vi "MapPositionSend.vi"(8 "error in (no error)":errorcluster caption="错误输入（无错误）", 10 "MapPosition":T1, 11 "CoordinatorState输入":refnum<class "CoordinatorState.lvclass">) -> (0 "error out":errorcluster caption="错误输出", 3 "Process State out":refnum<class "State Actor.lvclass">)   [LabVIEW 2014, in "States.lvlib" / "CoordinatorState.lvclass"]
uses:
  CoordinatorState.lvclass
  <vilib>/NI/Actors/State Actor/State Actor/State Actor.lvclass
  CoordinatorState.lvclass/CoordinatorState.ctl
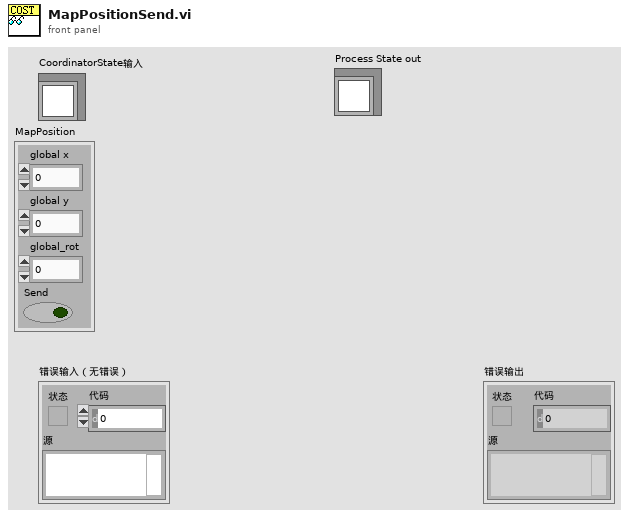
[diagram p1: front panel]
types:
  T1 = cluster{"global x":dbl, "global y":dbl, "global_rot":dbl, "Send":bool}
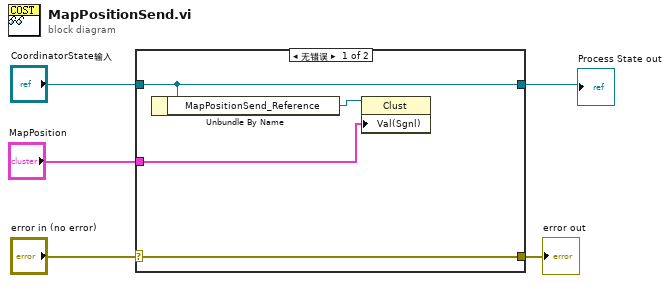
[diagram p0: block diagram]
diagram:
  n1 = case shown="无错误" "error in (no error)" {
    selector: "error in (no error)" -> [w9 w10]
    tunnel: [w9 w10] -> w4
    tunnel: [w8 w11] -> w1
    tunnel: "CoordinatorState输入" -> [w8 w11]
    tunnel: "MapPosition" -> [w6 _]
    frame No Error {
      n2 = Unbundle By Name(w8) -> ("MapPositionSend_Reference"=w7:refnum<vi>)
      n3 = property class="Clust"(reference=w7, "Val(Sgnl)"=w6) -> ()  [unwired: 1 in, 2 out]
    }
    frame Error {
    }
  }
  "error out" <- w4
  "Process State out" <- w1
